vi "RichToFlatnidaqmx_grpc_CfgImplicitTimingRequest.vi"(5 "OutputClusterType":T1, 11 "InputCluster":T4) -> (3 "OutputCluster":T1)   [LabVIEW 2021, in "NI DAQmx_server.lvlib"]
uses:
  NI DAQmx_server.lvlib
  nidaqmx_grpc_CfgImplicitTimingRequest.ctl
  nidevice_grpc_Session_session/nidevice_grpc_Session_session.lvclass
  nidaqmx_grpc_CfgImplicitTimingRequest_sample_mode_enum/nidaqmx_grpc_CfgImplicitTimingRequest_sample_mode_enum.lvclass
  nidevice_grpc_Session.ctl
  nidaqmx_grpc_CfgImplicitTimingRequest_Flat.ctl
  nidevice_grpc_Session_Flat.ctl
  nidaqmx_grpc_AcquisitionType.ctl
  nidevice_grpc_Session_session/nidevice_grpc_Session_session.lvclass/nidevice_grpc_Session_session.ctl
  nidaqmx_grpc_CfgImplicitTimingRequest_sample_mode_enum/nidaqmx_grpc_CfgImplicitTimingRequest_sample_mode_enum.lvclass/nidaqmx_grpc_CfgImplicitTimingRequest_sample_mode_enum.ctl
  nidevice_grpc_Session_session/Getname.vi
  nidevice_grpc_Session_session/Getid.vi
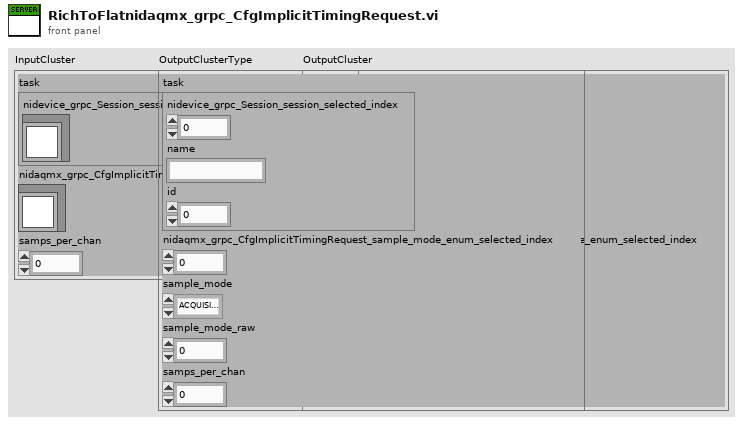
[diagram p1: front panel]
types:
  T1 = typedef "NI DAQmx_server.lvlib/nidaqmx_grpc_CfgImplicitTimingRequest_Flat.ctl" = cluster{"task":T2, "nidaqmx_grpc_CfgImplicitTimingRequest_sample_mode_enum_selected_index":i32, "sample_mode":T3, "sample_mode_raw":i32, "samps_per_chan":u64}
  T2 = typedef "NI DAQmx_server.lvlib/nidevice_grpc_Session_Flat.ctl" = cluster{"nidevice_grpc_Session_session_selected_index":i32, "name":string, "id":u32}
  T3 = typedef "NI DAQmx_server.lvlib/nidaqmx_grpc_AcquisitionType.ctl" = enum32{"ACQUISITION_TYPE_UNSPECIFIED", "ACQUISITION_TYPE_FINITE_SAMPS", "ACQUISITION_TYPE_CONT_SAMPS", "ACQUISITION_TYPE_HW_TIMED_SINGLE_POINT"}
  T4 = typedef "NI DAQmx_server.lvlib/nidaqmx_grpc_CfgImplicitTimingRequest.ctl" = cluster{"task":T5, "nidaqmx_grpc_CfgImplicitTimingRequest_sample_mode_enum":refnum<class "nidaqmx_grpc_CfgImplicitTimingRequest_sample_mode_enum.lvclass">, "samps_per_chan":u64}
  T5 = typedef "NI DAQmx_server.lvlib/nidevice_grpc_Session.ctl" = cluster{"nidevice_grpc_Session_session":refnum<class "nidevice_grpc_Session_session.lvclass">}
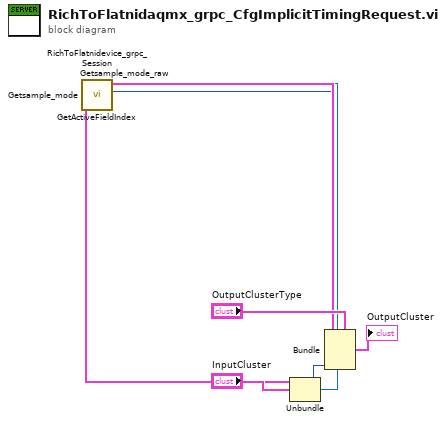
[diagram p0: block diagram]
diagram:
  n1 = Unbundle "Unbundle"("InputCluster") -> ("task"=w7:T5, "nidaqmx_grpc_CfgImplicitTimingRequest_sample_mode_enum"=w5:refnum<class "nidaqmx_grpc_CfgImplicitTimingRequest_sample_mode_enum.lvclass">, "samps_per_chan"=w1:u64)
  n2 = call "Getsample_mode_raw.vi"("OneOfTemplate in"=w5) -> ("Get_Val"=w2:i32)  [unwired: 8 in, 2 out]
  n3 = call "Getsample_mode.vi"("OneOfTemplate in"=w5) -> ("Get_Val"=w3:T3)  [unwired: 8 in, 2 out]
  n4 = call "GetActiveFieldIndex.vi"("OneOfTemplate in"=w5) -> ("Active Field Index"=w4:i32)  [unwired: 8 in, 2 out]
  n5 = call "RichToFlatnidevice_grpc_Session.vi"("InputCluster"=w7) -> ("OutputCluster"=w6:T2)  [unwired: 10 in]
  n6 = Bundle "Bundle"(cluster="OutputClusterType", "task"=w6, "nidaqmx_grpc_CfgImplicitTimingRequest_sample_mode_enum_selected_index"=w4, "sample_mode"=w3, "sample_mode_raw"=w2, "samps_per_chan"=w1) -> (→"OutputCluster":T1)
